vi "Camera setup acquisition.vi"(0 "Camera Parameters (important)":T4={"Exposure Time (sec)"=0.1, "EM CCD Gain"=230, "Readout Settings"={"Acquisition Mode"=enum."Single Scan", "Pixel Rate"=enum."EM CCD 1 Mhz 16 bits", "High Capacity?"=FALSE, "V Shift Speed (us/row)"=enum."4.33", "V Shift Amplitude"=enum."+1", "Preamp Gain"=enum."2", "Trigger Mode"=0, "Baseline offset"=0, "Baseline clamp"=TRUE}, "Image Size"={"H Bin"=1, "V Bin"=1, "Left"=1, "Top"=1, "Right"=512, "Bottom"=512}} {"Readout Settings"."Baseline offset" min=-1000 max=1000 step=100; "Readout Settings"."Trigger Mode" items=["Internal", "External"]; "EM CCD Gain" scale=1.0..300.0; "Exposure Time (sec)" scale=0.001..10.0 scale format="%#_1g"}) -> (14 "Image Size Out":T7={"H Bin"=1, "V Bin"=1, "Left"=1, "Top"=1, "Right"=512, "Bottom"=512} {"Top" min=4 max=2048 step=4; "Left" min=4 max=2048 step=4; "V Bin" min=1 max=2048 step=4; "H Bin" min=1 max=2048 step=4}, 15 "Continue with acq?":bool, 16 "Glimpse file properties":T1 {"Max Space Req'd. (Gb)" format="%.2f"}, 19 "Error Out (no error)":errorcluster)   [LabVIEW 2015]
doc: "This VI sets the hardware and Glimpse parameters for acquisition from the Cascade camera. If requested, shows a live video preview to allow setting of acquisition AOI and other camera parameters. When user presses \"GO\", vi exits leaving camera setup. Intended for use as a sub-vi, interactively or non-.\n\nLimitations: does not display current temperatures"
uses:
  h-nu-ixon/Laser type.ctt
  ixon camera/image size.ctl
  h-nu-ixon/Emission filters.ctl
  ixon ultra1024/HAL camera parameters important.ctt
  ixon ultra1024/ixon readout settings.ctl
  ixon ultra1024/andor acquisition mode.ctl
  Glimpse file parameters.ctt
  <vilib>/vision/Image Controls.llb/IMAQ Image.ctl
  camera globals.vi
  Autofocus Globals.vi
panel:
  in  "Continuous autofocus during\npreview?":bool caption="(CAUTION: use an\nemission filter that protects\ncamera from IR scatter!)"
  in  "Set to AOI":bool
  in  "Set to 512 x 300":bool
  in  "Set to Maximum":bool
  out "Actual Exposure Time (sec)":sgl format="%.4f"
  in  "Preview Shutters":T2[](array[typedef])
  in  "Preview emission filter":T3
  in  "Number of preview windows":i32=1
  in  "Go? (F)":bool
  in  "Quit":bool
  in  "Preview?":bool
  # "Information:"
  # "Parameters for non-interactive use"
  # "Camera: Andor iXon Ultra"
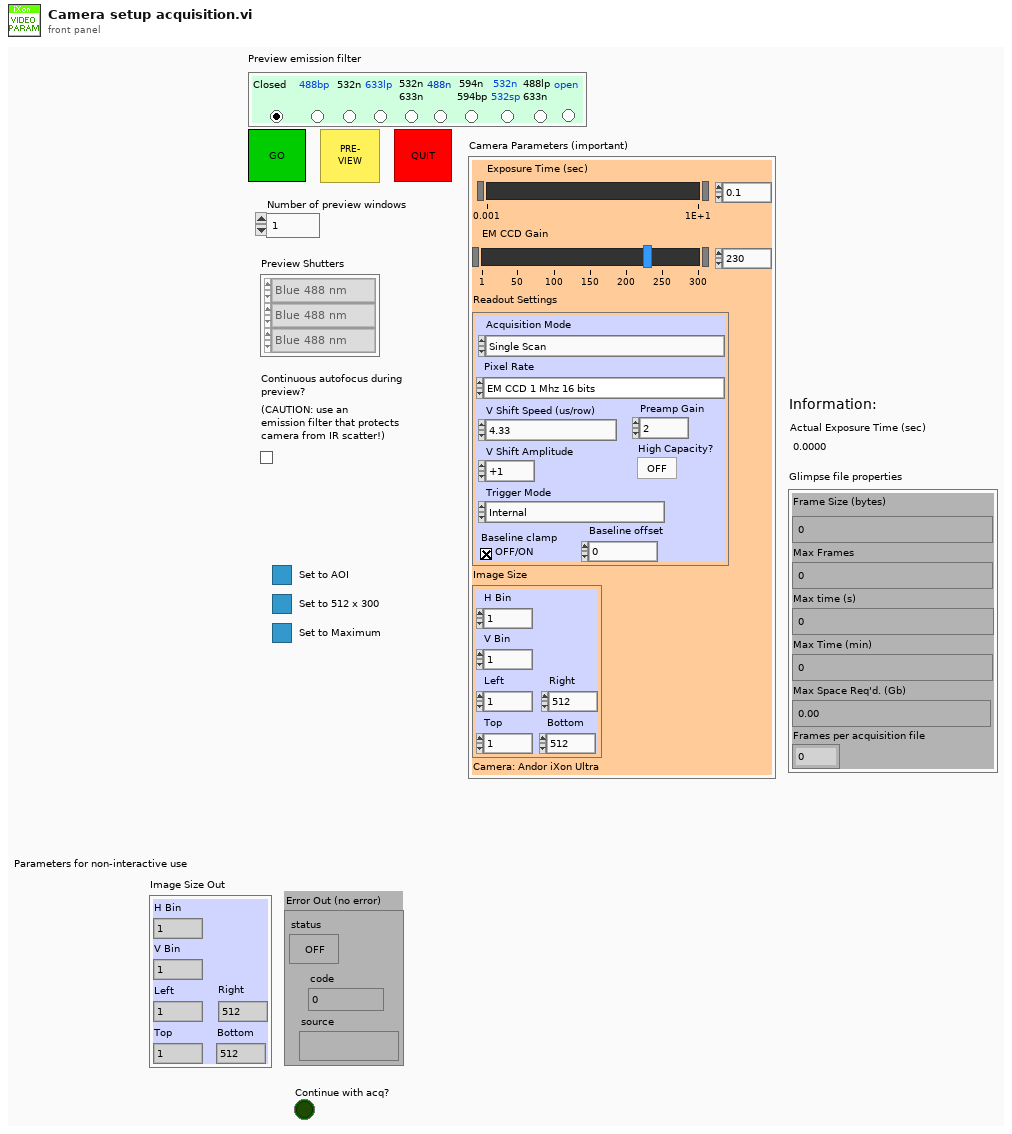
[diagram p1: front panel]
types:
  T1 = typedef "Glimpse file parameters.ctt" = cluster{"Frame Size (bytes)":u32, "Max Frames":u32, "Max time (s)":u32, "Max Time (min)":u32, "Max Space Req'd. (Gb)":dbl, "Frames per acquisition file":u32}
  T2 = typedef "Laser type.ctt" = enum16{"Blue 488 nm", "Green 532 nm", "Orange 594 nm", "Red 633 nm", "IR 780"}
  T3 = typedef "Emission filters.ctl" = enum32{" Closed ", "488bp ", "532n", "633lp ", "532n\n633n", "488n", "594n\n594bp", "532n\n532sp", "488lp\n633n", "open"}
  T4 = typedef "HAL camera parameters important.ctt" = cluster{"Exposure Time (sec)":sgl, "EM CCD Gain":u16, "Readout Settings":T5, "Image Size":cluster{"H Bin":i32, "V Bin":i32, "Left":i32, "Top":i32, "Right":i32, "Bottom":i32}}
  T5 = typedef "ixon readout settings.ctl" = cluster{"Acquisition Mode":T6, "Pixel Rate":enum16{"EM CCD 30 Mhz 16 bits", "EM CCD 20 Mhz 16 bits", "EM CCD 10 Mhz 16 bits", "EM CCD 1 Mhz 16 bits", "Standard CCD 1 Mhz 16 bits", "Standard CCD 0.1 Mhz 16 bits"}, "High Capacity?":bool, "V Shift Speed (us/row)":enum16{"0.6", "1.13 ", "2.2 ", "4.33"}, "V Shift Amplitude":enum16{"normal", "+1", "+2", "+3", "+4"}, "Preamp Gain":enum16{"1", "2", "3"}, "Trigger Mode":u32, "Baseline offset":i16, "Baseline clamp":bool}
  T6 = typedef "andor acquisition mode.ctl" = enum16{"(do not use)", "Single Scan", "Accumulate", "Kinetics", "Fast Kinetics", "Kinetics Run till Abort", "Frame Transfer", "Frame Transfer Run till Abort", "(do not use) ", "Time Delayed Integration"}
  T7 = typedef "image size.ctl" = cluster{"H Bin":i32, "V Bin":i32, "Left":i32, "Top":i32, "Right":i32, "Bottom":i32}
  T8 = typedef "IMAQ Image.ctl" = refnum<image>
  T9 = typedef "ROI Descriptor" = cluster{"Global Rectangle":i32[], "Contours":cluster{"ID":enum32{"External", "Internal"}, "Type":u32, "Coordinates":i32[]}[]}
  T10 = typedef "HAL camera properties.ctl" = cluster{"Head Model":string, "Serial number":i32, "Number of H pixels":i32, "Number of V pixels":i32, "Minimum temperature":i32, "Maximum temperature":i32}
  T11 = cluster{"H Bin":i32, "V Bin":i32, "Left":i32, "Top":i32, "Right":i32, "Bottom":i32}
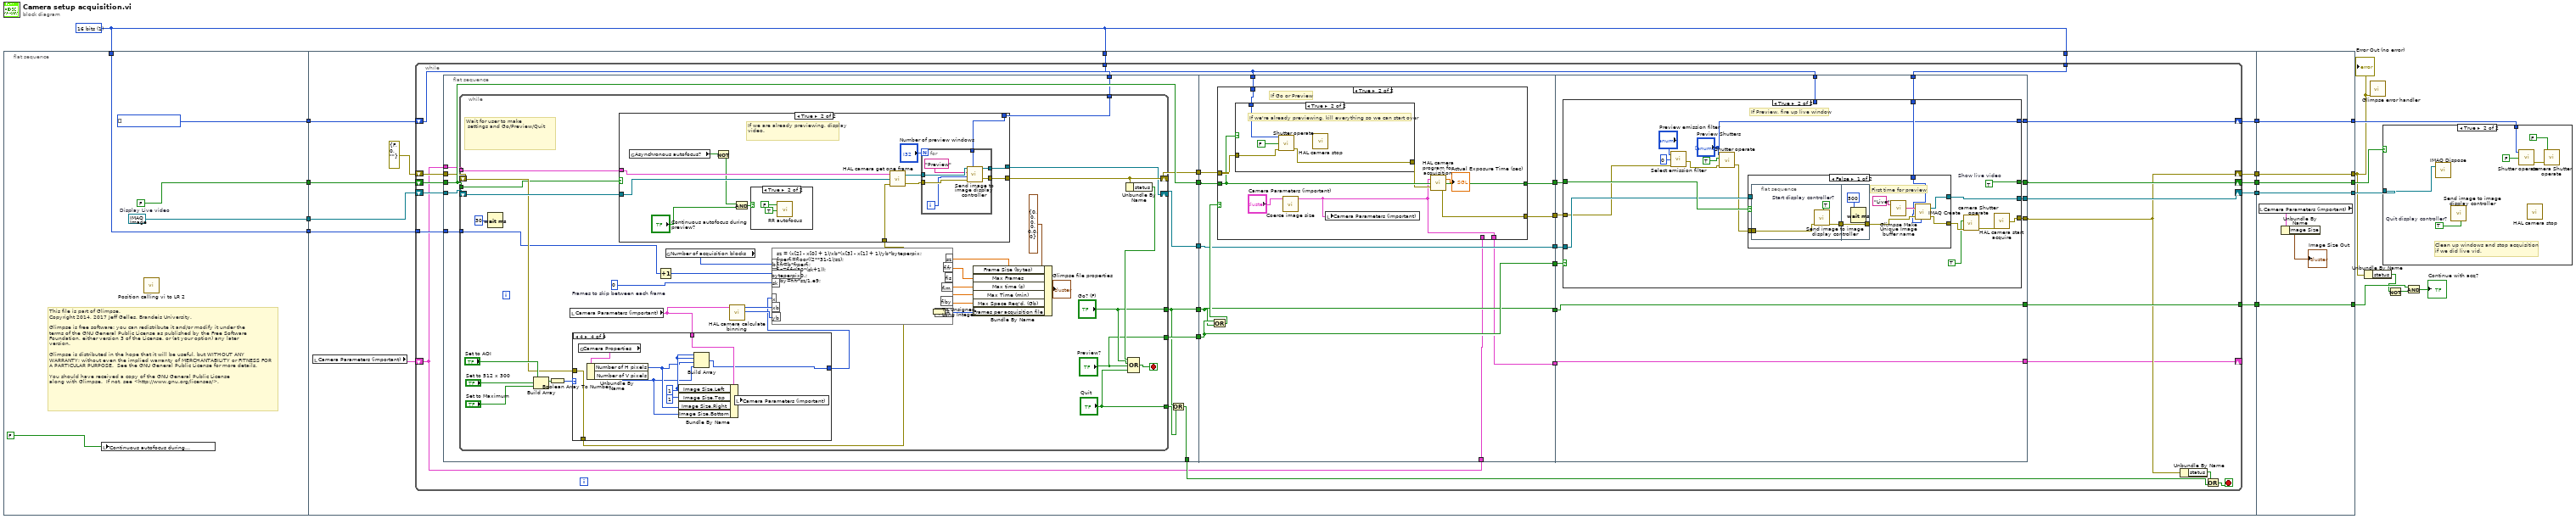
[diagram p0: block diagram]
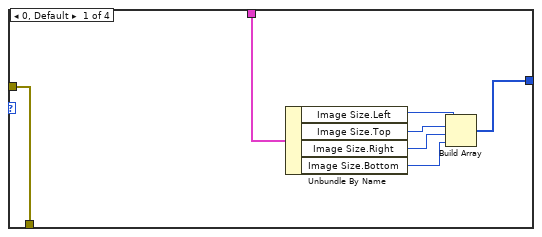
[diagram p4: hidden frame]
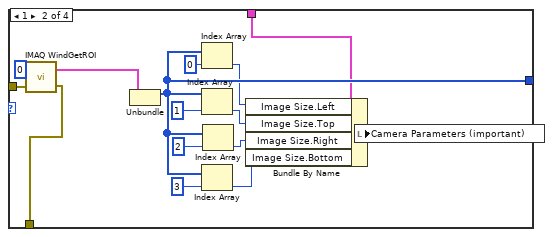
[diagram p5: hidden frame]
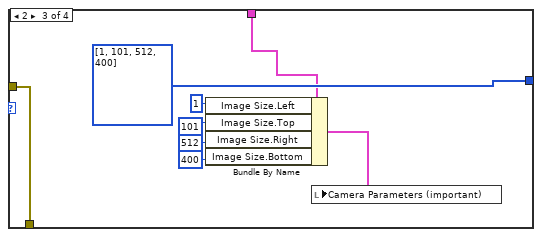
[diagram p6: hidden frame]
diagram:
  w11 = u32 1 items=["8 bits", "16 bits", "Float", "Complex", "RGB", "HSL"] ("Image Type")
  n1 = flat-sequence {
    tunnel: [w23] -> w16
    tunnel: [T8 refnum ("New Image")] -> w14
    tunnel: w11 -> [w20]
    tunnel: [w21] -> w10
    tunnel: [w20] -> w8
    tunnel: w16 -> [w36]
    tunnel: w14 -> [w32]
    tunnel: w11 -> [w30]
    tunnel: w11 -> [w29]
    tunnel: w10 -> [w28]
    tunnel: w8 -> [w26]
    tunnel: [w35] -> w7
    tunnel: [w34] -> w6
    tunnel: [w33] -> w5
    tunnel: [w31] -> w4
    tunnel: [w27] -> w3
    tunnel: [w252] -> w9
    tunnel: [w253] -> w13
    tunnel: [w254] -> w17
    tunnel: [w255] -> w2
    tunnel: [w256] -> w18
    tunnel: w7 -> [w256]
    tunnel: w6 -> [w255]
    tunnel: w5 -> [w254]
    tunnel: w4 -> [w253]
    tunnel: w3 -> [w252]
    frame #0 {
      w21 = T2[] [] items=["Blue 488 nm", "Green 532 nm", "Orange 594 nm", "Red 633 nm", "IR 780"] ("Preview Shutters")
      w23 = FALSE  # Display Live video
      # "This file is part of Glimpse. \nCopyright 2014, 2017 Jeff Gelles, Brandeis University.    \n\nGlimpse is free software: you can redistribute it and/or modify it under the \nterms of the GNU General Public License as published by the Free Software \nFoundation, either version 3 of the License, or (at your option) any later \nversion.\n\nGlimpse is distributed in the hope that it will be useful, but WITHOUT ANY \nWARRANTY; without even the implied warranty of MERCHANTABILITY or FITNESS FOR \nA PARTICULAR PURPOSE.  See the GNU General Public License for more details.\n\nYou should have received a copy of the GNU General Public License\nalong with Glimpse.  If not, see <http://www.gnu.org/licenses/>."
      n2 = local write "Continuous autofocus during\npreview?"(FALSE ("Continuous autofocus during\npreview? (CAUTION: use an\nemission filter that protects\ncamera from IR scatter!)")) -> ()
      n3 = call "Position calling vi to LR 2.vi"() -> ()  [unwired: 2 in, 4 out]
    }
    frame #1 {
      n4 = local read "Camera Parameters (important)"() -> (w24:T4)
      n5 = while {
        shift-right: [w62] -> w35
        shift-left: w36 -> [w64]
        shift-right: [w61] -> w31
        shift-left: w32 -> [w51]
        shift-right: [w40] -> w34
        shift-left: errorcluster {"status"=FALSE, "code"=0, "source"=""} ("error out") -> [w63]
        tunnel: [w60] -> w33
        tunnel: w30 -> [w45]
        tunnel: w29 -> [w44]
        shift-right: [w43] -> w27
        shift-left: w28 -> [w42]
        tunnel: w26 -> [w41]
        shift-right: [w38] -> _
        shift-left: w24 -> [w37]
        stop <- w50 stop-if-true
        n6 = flat-sequence {
          tunnel: w64 -> [w76]
          tunnel: [w76] -> w59
          tunnel: w51 -> [w75]
          tunnel: w63 -> [w74]
          tunnel: [w73] -> w58
          tunnel: [w70] -> w57
          tunnel: [w72] -> w56
          tunnel: [w69] -> w48
          tunnel: [w68] -> w47
          tunnel: w45 -> [w67]
          tunnel: w41 -> [w66]
          tunnel: w37 -> [w65]
          tunnel: w59 -> [w183]
          tunnel: [w180] -> w55
          tunnel: [w186] -> w54
          tunnel: w58 -> [w185]
          tunnel: w57 -> [w180]
          tunnel: w56 -> [w184]
          tunnel: [w184] -> w53
          tunnel: [w181] -> w52
          tunnel: w47 -> [w179]
          tunnel: [w179] -> w46
          tunnel: w42 -> [w178]
          tunnel: [w177] -> w39
          tunnel: w37 -> [w176]
          tunnel: w52 -> [w212]
          tunnel: [w211] -> w62
          tunnel: [w210] -> w61
          tunnel: [w209] -> w40
          tunnel: [w208] -> w60
          tunnel: w55 -> [w208]
          tunnel: w54 -> [w213]
          tunnel: w53 -> [w214]
          tunnel: w46 -> [w207]
          tunnel: w44 -> [w206]
          tunnel: [w205] -> w43
          tunnel: w42 -> [w204]
          tunnel: w39 -> [w203]
          tunnel: [w203] -> w38
          frame #0 {
            n7 = while {
              shift-left: w74 -> [w106]
              shift-right: [w101] -> w73
              tunnel: ["Go? (F)"] -> w70
              tunnel: w76 -> [w103]
              tunnel: ["Preview?"] -> w72
              tunnel: ["Quit"] -> w71
              shift-right: [w99] -> w68
              shift-left: w75 -> [w107]
              tunnel: w67 -> [w98]
              tunnel: w66 -> [w96]
              tunnel: w65 -> [w87]
              stop <- w88 stop-if-true
              w102 = u16 0  # Frames to skip between each frame
              # "Wait for user to make\n settings and Go/Preview/Quit"
              n8 = Wait (ms)(milliseconds to wait=u32 30) -> ()  [unwired: 1 out]
              n9 = Build Array("Set to AOI", "Set to 512 x 300", "Set to Maximum") -> (w112:bool[])
              n10 = Boolean Array To Number(Boolean array=w112) -> (number=w108:u32)
              n11 = local read "Camera Parameters (important)"() -> (w86:T4)
              n12 = case shown="4" w108 {
                tunnel: w106 -> [w143 w158 w166 w175]
                tunnel: [w137 w151 i32[] [1, 101, 512, 400] ("Global Rectangle") w168] -> w93
                tunnel: [w143 w156 w166 w175] -> w100
                tunnel: w86 -> [w138 w144 w159 w172]
                frame 0, Default {
                  n13 = Unbundle By Name(w138) -> ("Image Size.Left"=w139:i32, "Image Size.Top"=w140:i32, "Image Size.Right"=w141:i32, "Image Size.Bottom"=w142:i32)
                  n14 = Build Array(w139, w140, w141, w142) -> (w137:i32[])
                }
                frame 1 {
                  n15 = call "IMAQ WindGetROI"("Window Number (0...15)"=0, "error in (no error)"=w158) -> ("ROI Descriptor"=w157:T9, "error out"=w156:errorcluster)  [unwired: 3 out]
                  n16 = Unbundle(w157) -> ("Global Rectangle"=w151:i32[])  [unwired: 1 out]
                  n17 = Index Array(array=w151, index=0) -> (element=w149:i32)
                  n18 = Index Array(array=w151, index=1) -> (element=w148:i32)
                  n19 = Index Array(array=w151, index=3) -> (element=w146:i32)
                  n20 = Index Array(array=w151, index=2) -> (element=w147:i32)
                  n21 = Bundle By Name(cluster=w144, "Image Size.Left"=w149, "Image Size.Top"=w148, "Image Size.Right"=w147, "Image Size.Bottom"=w146) -> (w150:T4)
                  n22 = local write "Camera Parameters (important)"(w150) -> ()
                }
                frame 2 {
                  n23 = Bundle By Name(cluster=w159, "Image Size.Left"=1 ("Left"), "Image Size.Top"=101 ("Top"), "Image Size.Right"=512 ("Right"), "Image Size.Bottom"=400 ("Bottom")) -> (w163:T4)
                  n24 = local write "Camera Parameters (important)"(w163) -> ()
                }
                frame 4 {
                  w171 = 1 ("Left")
                  n25 = global read "camera globals.vi" "Camera Properties"() -> (w167:T10)
                  n26 = Unbundle By Name(w167) -> ("Number of H pixels"=w170:i32, "Number of V pixels"=w169:i32)
                  n27 = Bundle By Name(cluster=w172, "Image Size.Left"=w171, "Image Size.Top"=1 ("Top"), "Image Size.Right"=w170, "Image Size.Bottom"=w169) -> (w174:T4)
                  n28 = Build Array(w171, w171, w170, w169) -> (w168:i32[])
                  n29 = local write "Camera Parameters (important)"(w174) -> ()
                }
              }
              n30 = case shown="True" w103 {
                tunnel: w107 -> [w113 w126]
                tunnel: [w114 w124] -> w101
                tunnel: w100 -> [w114 w127]
                tunnel: [w113 w125] -> w99
                tunnel: w98 -> [_ w120]
                tunnel: w87 -> [_ w119]
                frame False {
                }
                frame True {
                  # "If we are already previewing, display video."
                  n31 = global read "Autofocus Globals.vi" "Asynchronous autofocus?"() -> (w118:bool)
                  n32 = Not(x=w118) -> (.not. x?=w117:bool)
                  n33 = And(x=w117, y="Continuous autofocus during\npreview?") -> (x .and. y?=w115:bool)
                  n34 = case shown="True" w115 {
                    frame False {
                    }
                    frame True {
                      n35 = call "RR autofocus.vi"("Close camera shutter during autofocus?"=FALSE, "Close laser shutter when autofocus is done?"=TRUE) -> ()  [unwired: 5 in, 1 out]
                    }
                  }
                  n36 = call "HAL camera get one frame.vi"("error in"=w127, "New Image"=w126, "Camera Parameters (important)"=w119) -> ("error out"=w123:errorcluster, "Image Out"=w121:T8)
                  n37 = for {
                    N: "Number of preview windows" -> [_]
                    tunnel: [w136] -> w125
                    tunnel: [w135] -> w124
                    tunnel: w123 -> [w134]
                    tunnel: w121 -> [w133]
                    tunnel: w120 -> [w130]
                    i -> [w131]
                    n38 = call "Send image to image display controller.vi"("Image"=w133, "Window Title"="Preview" ("Window Title\n(Window only)"), "Window Number"=w131, "error in"=w134, "Image Type"=w130) -> ("Image Out"=w136:T8, "error out"=w135:errorcluster)  [unwired: 2 in, 2 out]
                  }
                }
              }
              n39 = Increment(x=w96) -> (x+1=w97:u32)
              n40 = global read "camera globals.vi" "Number of acquisition blocks"() -> (w85:i8)
              n41 = call "HAL camera calculate binning.vi"("Camera Parameters (important)"=w86) -> ("V Bin"=w94:i32, "H Bin"=w95:i32)  [unwired: 9 in]
              n42 = formula code="sz = (x[2] - x[0] + 1)/xb*(x[3] - x[1] + 1)/yb*byteperpix;\nfrperfi=floor((2**31-1)/sz);\nfifr=b*frperfi;\nfis=fifr/(30*(sk+1));\nfim=fis/60.;\nfiby=fifr*sz/1.e9;"("x"=w93, "b"=w85, "sk"=w102, "xb"=w95, "yb"=w94, "byteperpix"=w97) -> ("sz"=w78:dbl, "fifr"=w77:dbl, "fis"=w79:dbl, "fim"=w80:dbl, "fiby"=w81:dbl, "frperfi"=w104:dbl)
              n43 = To Unsigned Long Integer(number=w104) -> (unsigned 32bit integer=w82:u32)
              n44 = Bundle By Name(cluster=T1 {"Frame Size (bytes)"=0, "Max Frames"=0, "Max time (s)"=0, "Max Time (min)"=0, "Max Space Req'd. (Gb)"=0.0, "Frames per acquisition file"=0} ("Glimpse file properties"), "Frame Size (bytes)"=w78, "Max Frames"=w77, "Max time (s)"=w79, "Max Time (min)"=w80, "Max Space Req'd. (Gb)"=w81, "Frames per acquisition file"=w82) -> (→"Glimpse file properties":T1)
              n45 = Unbundle By Name(w101) -> ("status"=w92:bool)
              n46 = Compound Arithmetic op=OR(w92, "Go? (F)", "Preview?", "Quit") -> (w88:bool)
            }
            n47 = Or(x=w70, y=w71) -> (x .or. y?=w69:bool)
          }
          frame #1 {
            n48 = Or(x=w184, y=w180) -> (x .or. y?=w182:bool)
            n49 = case shown="True" w182 {
              tunnel: [w189 w192] -> w186
              tunnel: w185 -> [w189 w196]
              tunnel: w183 -> [w188 w197]
              tunnel: [w188 w197] -> w181
              tunnel: w178 -> [_ w195]
              tunnel: [w187 w190] -> w177
              tunnel: w176 -> [w187 _]
              frame False {
              }
              frame True {
                # "If Go or Preview"
                n50 = case shown="True" w197 {
                  tunnel: w196 -> [w198 w199]
                  tunnel: [w198 w201] -> w194
                  tunnel: w195 -> [_ w200]
                  frame False {
                  }
                  frame True {
                    # "If we're already previewing, kill everything so we can start over"
                    n51 = call "Shutter operate.vi"("Shutters"=w200, 2:FALSE, "error in"=w199) -> ("error out"=w201:errorcluster)  [unwired: 5 out]
                    n52 = call "HAL camera stop.vi"() -> ()  [unwired: 1 out]
                  }
                }
                n53 = call "Coerce image size.vi"("Camera Parameters (important) in"="Camera Parameters (important)") -> ("Camera Parameters (important) out"=w190:T4)  [unwired: 10 in]
                n54 = local write "Camera Parameters (important)"(w190) -> ()
                n55 = call "HAL camera program for acquisition.vi"("error in"=w194, "Camera Parameters (important)"=w190) -> ("error out"=w192:errorcluster, "Actual Exposure Time (sec)"=→"Actual Exposure Time (sec)":sgl)
              }
            }
          }
          frame #2 {
            n56 = case shown="True" w214 {
              tunnel: w213 -> [w217 w220]
              tunnel: [w218 w234] -> w211
              tunnel: w212 -> [w218 w232]
              tunnel: [w216 w233] -> w210
              tunnel: [w217 w225] -> w209
              tunnel: w207 -> [w216 w231]
              tunnel: w206 -> [_ w230]
              tunnel: [w215 "Preview Shutters"] -> w205
              tunnel: w204 -> [w215 _]
              frame False {
              }
              frame True {
                w234 = TRUE  # Show live video
                # "If Preview, fire up live window"
                n57 = call "Select emission filter.vi"("Emission filter"="Preview emission filter", "Time to wait\nafter filter change\n(ms)"=u32 0 ("Time to wait\nafter filter change\n(ms)"), "error in"=w220) -> ("error out"=w221:errorcluster)  [unwired: 3 out]
                n58 = call "Shutter operate.vi"("Shutters"="Preview Shutters", 2:TRUE, "error in"=w221) -> ("error out"=w228:errorcluster)  [unwired: 5 out]
                n59 = case shown="False" w232 {
                  tunnel: [w242 w248] -> w226
                  tunnel: [w239 w249] -> w233
                  tunnel: w231 -> [_ w249]
                  tunnel: w230 -> [w235 _]
                  tunnel: w228 -> [w238 w248]
                  frame False {
                    # "First time for preview"
                    n60 = flat-sequence {
                      tunnel: w238 -> [w244]
                      tunnel: [w243] -> w236
                      tunnel: [w247] -> w237
                      tunnel: w236 -> [w247]
                      frame #0 {
                        w245 = TRUE  # Start display controller?
                        n61 = call "Send image to image display controller.vi"("error in"=w244, "Start display controller?"=w245) -> ("error out"=w243:errorcluster)  [unwired: 5 in, 3 out]
                      }
                      frame #1 {
                        n62 = Wait (ms)(milliseconds to wait=u32 500) -> ()  [unwired: 1 out]
                      }
                    }
                    n63 = call "Glimpse Make Unique Image buffer name.vi"("Buffer  base name"="Live" ("Image Name")) -> ("Image Name"=w240:string)  [unwired: 1 in]
                    n64 = call "IMAQ Create"("Image Name"=w240, "Image Type"=w235, "error in (no error)"=w237) -> ("New Image"=w239:T8, "error out"=w242:errorcluster)  [unwired: 1 in, 1 out]
                  }
                  frame True {
                  }
                }
                n65 = call "camera Shutter operate.vi"("Open?"=TRUE, "error in"=w226) -> ("error out"=w224:errorcluster)  [unwired: 6 out]
                n66 = call "HAL camera start acquire.vi"("error in"=w224) -> ("error out"=w225:errorcluster)
              }
            }
          }
        }
        n67 = Unbundle By Name(w40) -> ("status"=w49:bool)
        n68 = Or(x=w49, y=w48) -> (x .or. y?=w50:bool)
      }
    }
    frame #2 {
      n69 = local read "Camera Parameters (important)"() -> (w251:T4)
      n70 = Unbundle By Name(w251) -> ("Image Size"=→"Image Size Out":T11)
    }
  }
  n71 = Unbundle By Name(w2) -> ("status"=w12:bool)
  n72 = call "Glimpse error handler.vi"("error in"=w2) -> ()  [unwired: 1 in, 6 out]
  n73 = case shown="True" w18 {
    tunnel: w13 -> [_ w262]
    tunnel: w9 -> [_ w260]
    frame False {
    }
    frame True {
      w259 = TRUE  # Quit display controller?
      # "Clean up windows and stop acquisition\nif we did live vid."
      n74 = call "IMAQ Dispose"("Image"=w262) -> ()  [unwired: 2 in, 4 out]
      n75 = call "Send image to image display controller.vi"("Quit display controller?"=w259) -> ()  [unwired: 6 in, 4 out]
      n76 = call "Shutter operate.vi"("Shutters"=w260, 2:FALSE) -> ("error out"=w257:errorcluster)  [unwired: 1 in, 5 out]
      n77 = call "HAL camera stop.vi"() -> ()  [unwired: 1 out]
      n78 = call "camera Shutter operate.vi"("Open?"=FALSE, "error in"=w257) -> ()  [unwired: 7 out]
    }
  }
  n79 = Not(x=w12) -> (.not. x?=w15:bool)
  n80 = And(x=w17, y=w15) -> (x .and. y?=→"Continue with acq?":bool)
  "Error Out (no error)" <- w2
